vi "Initialize oscilloscope.vi"(7 "Serial Configuration":T1, 8 "error in":errorcluster, 9 "Reset? (T: Yes)":bool, 10 "ID Query? (T: Yes)":bool, 11 "Module ID":i32=-1) -> (0 "error out":errorcluster)   [LabVIEW 2020, in "Oscilloscope.lvlib"]
doc: "Initialize the oscilloscope\n_____\nCreated using DQMH Event Scripter 6.0.0.122."
uses:
  Oscilloscope.lvlib
  Initialize oscilloscope Argument--cluster.ctl
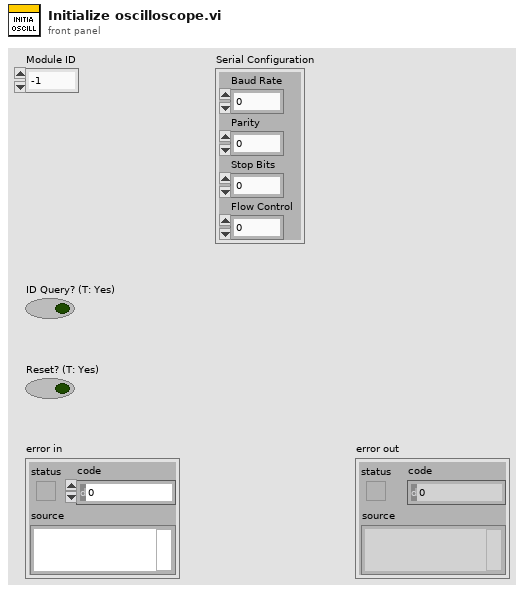
[diagram p1: front panel]
types:
  T1 = cluster{"Baud Rate":u32, "Parity":u16, "Stop Bits":u16, "Flow Control":u16}
  T2 = typedef "Oscilloscope.lvlib/Initialize oscilloscope Argument--cluster.ctl" = cluster{"Module ID":i32, "ID Query? (T: Yes)":bool, "Reset? (T: Yes)":bool, "Serial Configuration":cluster{"Baud Rate":u32, "Parity":u16, "Stop Bits":u16, "Flow Control":u16}}
  T3 = typedef "Oscilloscope.lvlib/Request Events--cluster.ctl" = cluster{"Stop Module":refnum<user-event>, "Show Panel":refnum<user-event>, "Hide Panel":refnum<user-event>, "Show Diagram":refnum<user-event>, "Get Module Execution Status":refnum<user-event>, "Set COM Port":refnum<user-event>, "Initialize OSC":refnum<user-event>, "Close":refnum<user-event>, "Autosetup":refnum<user-event>, "Configure Channel":refnum<user-event>, "Read Waveform":refnum<user-event>, "Read Measurement":refnum<user-event>, "Read Measurement 2 Channels":refnum<user-event>, "Reset":refnum<user-event>, "Read Waveform RP":refnum<user-event>, "Initialize oscilloscope":refnum<user-event>}
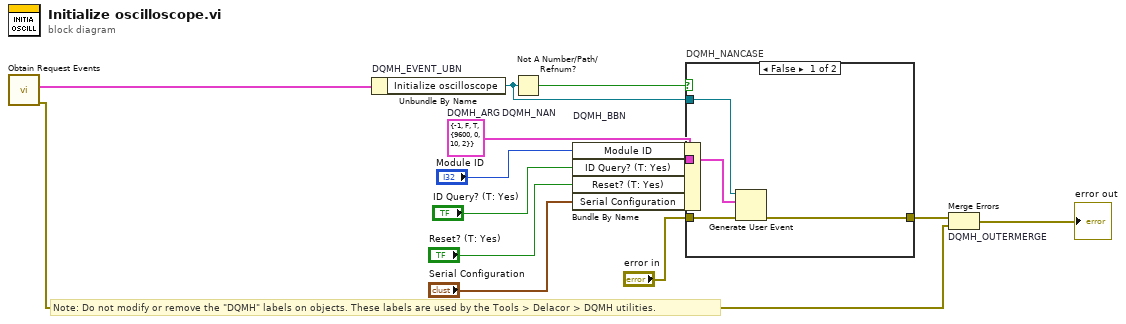
[diagram p0: block diagram]
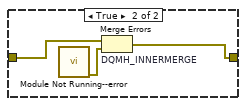
[diagram p2: hidden frame]
diagram:
  w7 = T2 {"Module ID"=-1, "ID Query? (T: Yes)"=FALSE, "Reset? (T: Yes)"=TRUE, "Serial Configuration"={"Baud Rate"=9600, "Parity"=0, "Stop Bits"=10, "Flow Control"=2}}  # DQMH_ARG
  # "Note: Do not modify or remove the \"DQMH\" labels on objects. These labels are used by the Tools > Delacor > DQMH utilities."
  n1 = call "Obtain Request Events.vi"() -> ("error out"=w5:errorcluster, "Oscilloscope Request Events"=w4:T3)  [unwired: 10 in]
  n2 = Unbundle By Name "DQMH_EVENT_UBN"(w4) -> ("Initialize oscilloscope"=w9:refnum<user-event>)
  n3 = Not A Number/Path/Refnum? "DQMH_NAN"(number/path/refnum=w9) -> (NaN/Path/Refnum?=w10:bool)
  n4 = Bundle By Name "DQMH_BBN"(cluster=w7, "Module ID"="Module ID", "ID Query? (T: Yes)"="ID Query? (T: Yes)", "Reset? (T: Yes)"="Reset? (T: Yes)", "Serial Configuration"="Serial Configuration") -> (w11:T2)
  n5 = case "DQMH_NANCASE" shown="False" w10 {
    tunnel: "error in" -> [w17 w20]
    tunnel: [w16 w19] -> w8
    tunnel: w9 -> [w15 _]
    tunnel: w11 -> [w14 _]
    frame False {
      n6 = Generate User Event(user event=w15, event data cluster=w14, error in=w17) -> (error out=w16:errorcluster)  [unwired: 1 in, 1 out]
    }
    frame True {
      n7 = call "Module Not Running--error.vi"() -> ("error out"=w18:errorcluster)  [unwired: 11 in]
      n8 = Merge Errors "DQMH_INNERMERGE"(w20, w18) -> (w19:errorcluster)
    }
  }
  n9 = Merge Errors "DQMH_OUTERMERGE"(w8, w5) -> (→"error out":errorcluster)
